vi "delay.vi"(7 "Delay Settings":T1 {"Wet/Dry" scale=0.0..1.0}, 9 "Audio R In":dbl[](array[numeric]), 11 "Audio L In":dbl[](array[numeric])) -> (1 "Audio R Out":dbl[](array[numeric]), 3 "Audio L Out":dbl[](array[numeric]))   [LabVIEW 2014]
uses:
  Controls/Delay Controls.ctl
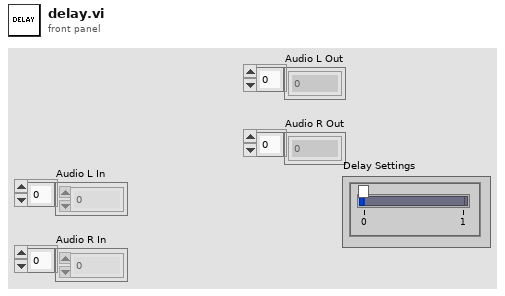
[diagram p1: front panel]
types:
  T1 = typedef "Delay Controls.ctl" = cluster{"Wet/Dry":dbl}
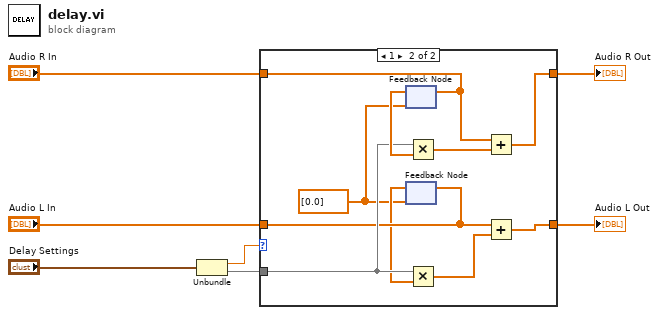
[diagram p0: block diagram]
diagram:
  n1 = Unbundle("Delay Settings") -> (w2:dbl, w1)
  n2 = case shown="1" w2 {
    tunnel: w1 -> [_ w16]
    tunnel: "Audio L In" -> [w9 w13]
    tunnel: [w9 w15] -> w4
    tunnel: "Audio R In" -> [w8 w19]
    tunnel: [w8 w14] -> w5
    frame 0, Default {
    }
    frame 1 {
      w10 = dbl[] [0.0] ("AudioIn/Left (N Samples)")
      n3 = feedback #1(w10) -> (w18:dbl[])
      n4 = feedback-in #1(w19) -> ()
      n5 = feedback #2(w10) -> (w11:dbl[])
      n6 = feedback-in #2(w13) -> ()
      n7 = Multiply(x=w16, y=w18) -> (x*y=w17:dbl[])
      n8 = Multiply(x=w16, y=w11) -> (x*y=w12:dbl[])
      n9 = Add(x=w19, y=w17) -> (x+y=w14:dbl[])
      n10 = Add(x=w13, y=w12) -> (x+y=w15:dbl[])
    }
  }
  "Audio R Out" <- w5
  "Audio L Out" <- w4
